vi "Configure Pulse.vi"(7 "Pulse Width (5E-5 seconds)":dbl=5e-05, 8 "error in (no error)":errorcluster, 9 "Pulse Delay (0 seconds)":dbl, 10 "Channel (0: Channel 1)":i32(ring) items=["Channel 1", "Channel 2"], 11 "VISA resource name":refnum<visa-resource-name>) -> (0 "error out":errorcluster, 3 "VISA resource name out":refnum<visa-resource-name>)   [LabVIEW 2020, in "Agilent B2900 Series.lvlib"]
doc: "Change settings for pulse mode."
uses:
  Agilent B2900 Series.lvlib
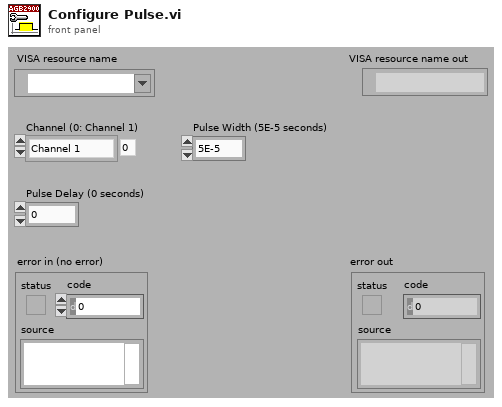
[diagram p1: front panel]
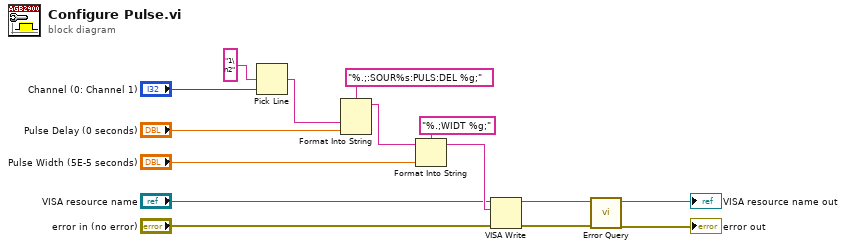
[diagram p0: block diagram]
diagram:
  n1 = Pick Line(multi-line string="1\n2" ("string (\"\")"), line index="Channel (0: Channel 1)") -> (output string=w1:string)  [unwired: 1 in]
  n2 = Format Into String(format string="%.;:SOUR%s:PULS:DEL %g;", w1, "Pulse Delay (0 seconds)") -> (resulting string=w13:string)  [unwired: 2 in, 1 out]
  n3 = Format Into String(format string="%.;WIDT %g;", initial string=w13, "Pulse Width (5E-5 seconds)") -> (resulting string=w10:string)  [unwired: 1 in, 1 out]
  n4 = VISA Write(VISA resource name="VISA resource name", write buffer=w10, error in (no error)="error in (no error)") -> (VISA resource name out=w7:refnum<visa-resource-name>, error out=w6:errorcluster)  [unwired: 1 out]
  n5 = call "Error Query.vi"("error in (no error)"=w6, "VISA resource name"=w7) -> ("error out"=→"error out":errorcluster, "VISA resource name out"=→"VISA resource name out":refnum<visa-resource-name>)  [unwired: 6 in, 2 out]
